vi "RawToScaled.vi"(8 "error in (no error)":errorcluster, 10 "RAW":dbl, 11 "PiecedLinearScale in":refnum<class "Scale_PiecedLinear.lvclass">) -> (0 "error out":errorcluster, 2 "Scaled":dbl, 3 "PiecedLinearScale out":refnum<class "Scale_PiecedLinear.lvclass">)   [LabVIEW 2019, in "Scale_PiecedLinear.lvclass"]
uses:
  Scale_PiecedLinear.lvclass
  Scale_PiecedLinear.lvclass/Scale_PiecedLinear.ctl
  <vilib>/gmath/NI_Gmath.lvlib
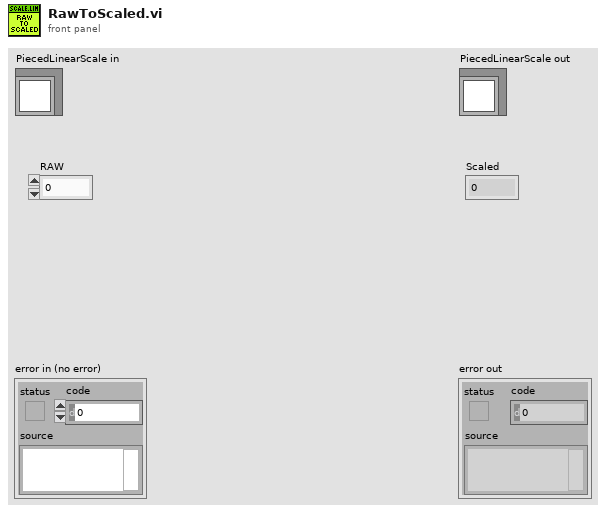
[diagram p1: front panel]
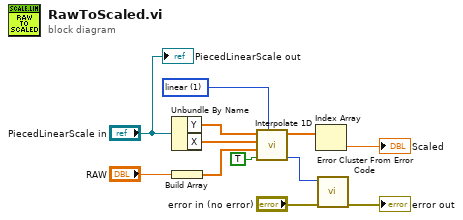
[diagram p0: block diagram]
diagram:
  w9 = 1 items=["nearest", "linear", "spline", "cubic Hermite", "Lagrange"] ("method")
  n1 = Unbundle By Name("PiecedLinearScale in") -> ("Y"=w8:dbl[], "X"=w11:dbl[])
  n2 = Build Array("RAW") -> (w6:dbl[])
  n3 = call <vilib>:"Interpolate 1D.vi"("method"=w9, "X is monotonic"=TRUE, "xi"=w6, "X"=w11, "Y"=w8) -> ("error"=w3:i32, "yi"=w5:dbl[])  [unwired: 4 in, 1 out]
  n4 = Index Array(array=w5) -> (element=→"Scaled":dbl)  [unwired: 1 in]
  n5 = call <vilib>:"Error Cluster From Error Code.vi"("error in (no error)"="error in (no error)", "error code (0)"=w3) -> ("error out"=→"error out":errorcluster)  [unwired: 7 in]
  "PiecedLinearScale out" <- "PiecedLinearScale in"
